vi "Rotate Two Files.vi"() -> ()   [LabVIEW 2021]
uses:
  6c21c491-3613-49b9-8739-58848ace7e6b.vi
  9d677228-37d7-4fae-91d8-cc659d765936.vi
  6babdee7-8c0c-47d0-81fc-a19b133f3013.vi
  911cfe7f-2ed1-4032-abb0-88a2fbac1f55.vi
panel:
  in  "Reverse File 2":bool
  in  "Averaging":dbl(slide) scale=1.0..1000.0
  in  "number of header lines":i32
  in  "Numeric":dbl step=5e-06 format="%.2e"
  out "X & Y 3":dbl[](graph)
  out "Array":sgl[](array[numeric]) format="%.2f"
  in  "Save":bool
  out "X & Y 2":dbl[][](graph)
  in  "CH2 File 1":sgl(slide) step=0.5 scale=-180.0..180.0
  in  "CH1 File 2":sgl(slide) step=0.1 scale=-180.0..180.0
  in  "CH2 File 2":sgl(slide) step=0.5 scale=-180.0..180.0
  in  "Channel 1 Y":i32=3
  in  "Channel 2 Y":i32=5
  in  "Channel 2 X":i32=4
  in  "Channel 1  X":i32=2
  out "X & Y":dbl[][](graph)
  in  "Phase OK":bool
  in  "CH1 File 1":sgl(slide) step=0.1 scale=-180.0..180.0
  in  "Input file 2":path
  in  "Data Source":T1(ring)
  in  "Input file 1":path
  # "ADD"
  # "ADD"
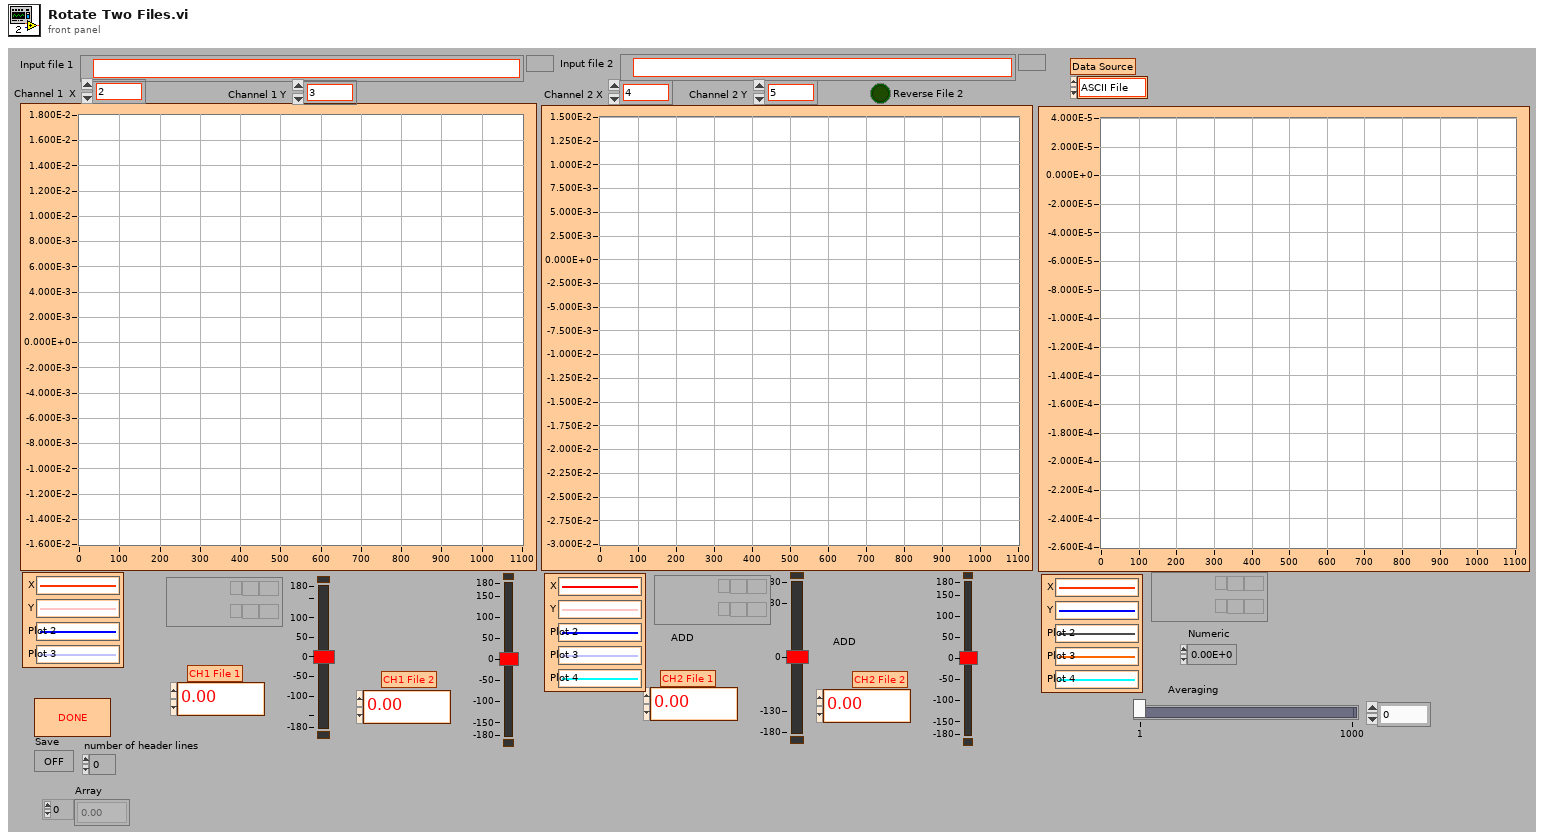
[diagram p1: front panel]
types:
  T1 = enum16{"ASCII File", "BinH File", "BinW File", "BINARY File"}
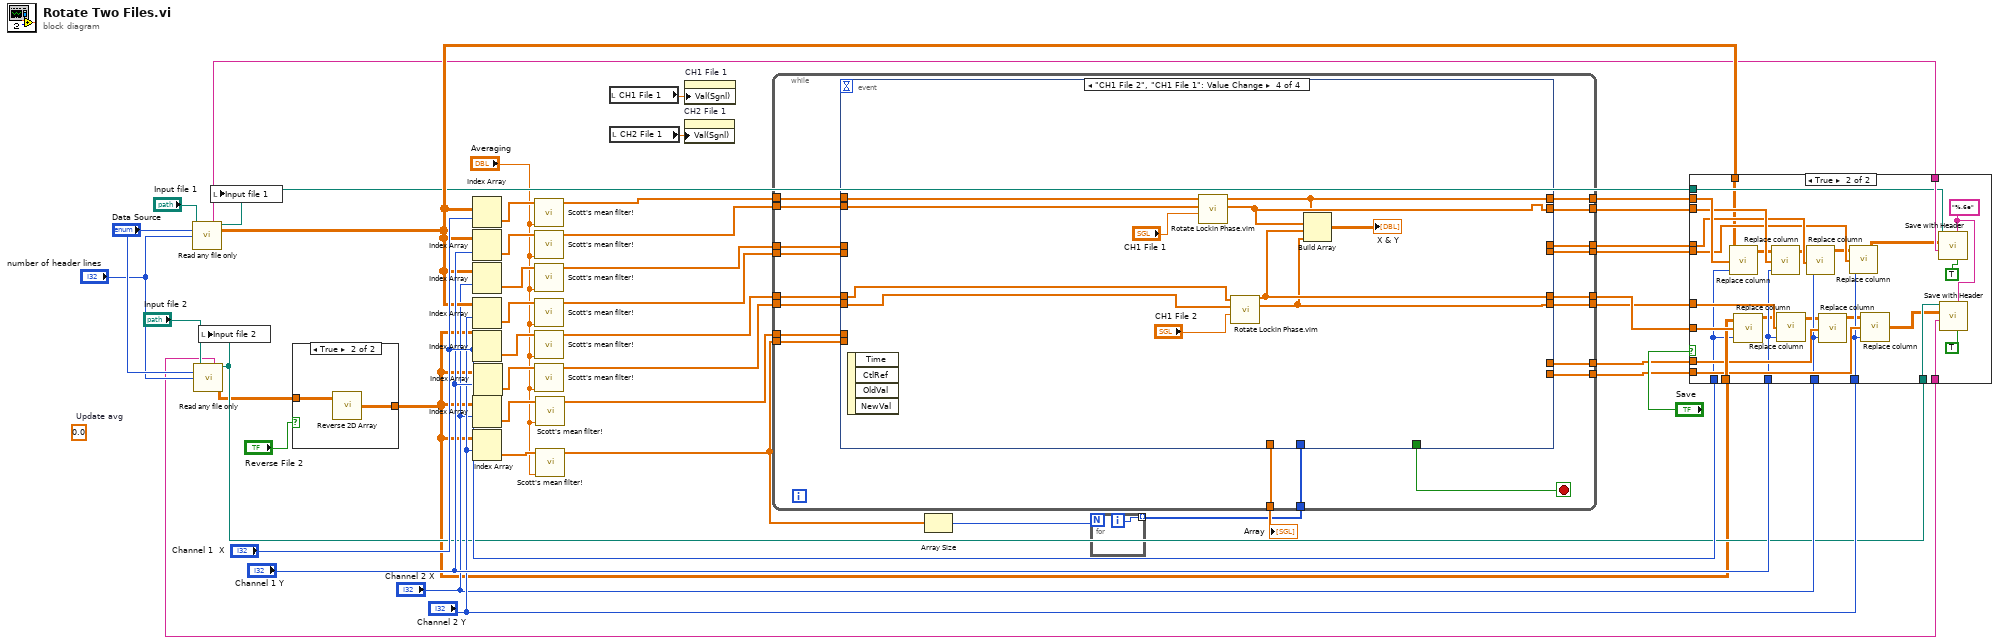
[diagram p0: block diagram]
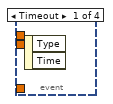
[diagram p3: hidden frame]
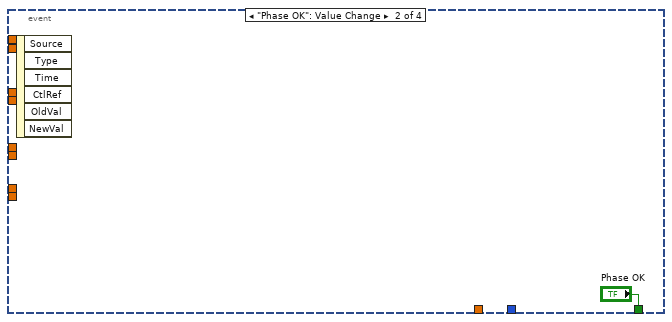
[diagram p4: hidden frame]
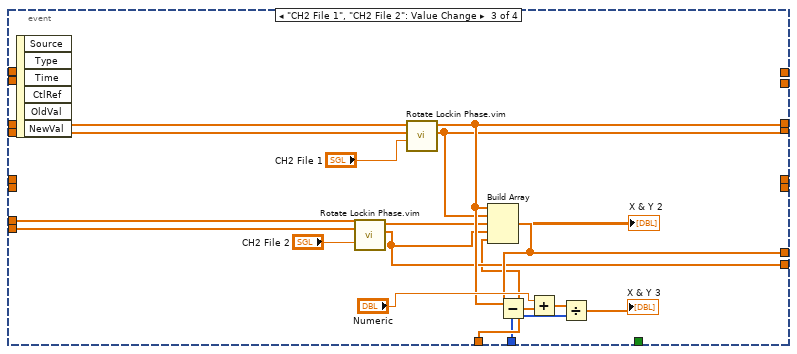
[diagram p5: hidden frame]
diagram:
  (unwired) 0.0  # Update avg
  n1 = call "Read any file only.vi"("Input file path"="Input file 1", "Data File Type"="Data Source", "number of header lines"="number of header lines") -> ("Header"=w26:string, "Actual input file path"=w24:path, "all rows"=w38:sgl[][])  [unwired: 6 in, 4 out]
  n2 = call "Read any file only.vi"("Input file path"="Input file 2", "Data File Type"="Data Source", "number of header lines"="number of header lines") -> ("Header"=w25:string, "Actual input file path"=w22:path, "all rows"=w2:sgl[][])  [unwired: 6 in, 4 out]
  n3 = local write "Input file 2"(w22) -> ()
  n4 = local write "Input file 1"(w24) -> ()
  n5 = case shown="True" "Reverse File 2" {
    tunnel: w2 -> [w48 w50]
    tunnel: [w48 w49] -> w1
    frame False {
    }
    frame True {
      n6 = call "Reverse 2D Array.vi"("Input array"=w50) -> ("Output Array"=w49:dbl[][])  [unwired: 1 in]
    }
  }
  n7 = Index Array(array=w38, index (row)="Channel 1  X") -> (element=w44:sgl[])  [unwired: 1 in]
  n8 = Index Array(array=w38, index (row)="Channel 1 Y") -> (element=w20:sgl[])  [unwired: 1 in]
  n9 = Index Array(array=w38, index (row)="Channel 2 X") -> (element=w18:sgl[])  [unwired: 1 in]
  n10 = Index Array(array=w38, index (row)="Channel 2 Y") -> (element=w16:sgl[])  [unwired: 1 in]
  n11 = Index Array(array=w1, index (row)="Channel 1  X") -> (element=w14:dbl[])  [unwired: 1 in]
  n12 = Index Array(array=w1, index (row)="Channel 2 X") -> (element=w10:dbl[])  [unwired: 1 in]
  n13 = Index Array(array=w1, index (row)="Channel 2 Y") -> (element=w8:dbl[])  [unwired: 1 in]
  n14 = Index Array(array=w1, index (row)="Channel 1 Y") -> (element=w12:dbl[])  [unwired: 1 in]
  n15 = call "Scott's mean filter!.vi"("window size"="Averaging", "input"=w44) -> ("output"=w21:dbl[])  [unwired: 9 out]
  n16 = call "Scott's mean filter!.vi"("window size"="Averaging", "input"=w20) -> ("output"=w19:dbl[])  [unwired: 9 out]
  n17 = call "Scott's mean filter!.vi"("window size"="Averaging", "input"=w18) -> ("output"=w17:dbl[])  [unwired: 9 out]
  n18 = call "Scott's mean filter!.vi"("window size"="Averaging", "input"=w16) -> ("output"=w15:dbl[])  [unwired: 9 out]
  n19 = call "Scott's mean filter!.vi"("window size"="Averaging", "input"=w14) -> ("output"=w13:dbl[])  [unwired: 9 out]
  n20 = call "Scott's mean filter!.vi"("window size"="Averaging", "input"=w12) -> ("output"=w11:dbl[])  [unwired: 9 out]
  n21 = call "Scott's mean filter!.vi"("window size"="Averaging", "input"=w10) -> ("output"=w9:dbl[])  [unwired: 9 out]
  n22 = call "Scott's mean filter!.vi"("window size"="Averaging", "input"=w8) -> ("output"=w7:dbl[])  [unwired: 9 out]
  n23 = local read "CH1 File 1"() -> (w4:sgl)
  n24 = local read "CH2 File 1"() -> (w5:sgl)
  n25 = property on="CH2 File 1" class="Slide (strict)"("Val(Sgnl)"=w5) -> ()  [unwired: 2 in, 2 out]
  n26 = property on="CH1 File 1" class="Slide (strict)"("Val(Sgnl)"=w4) -> ()  [unwired: 2 in, 2 out]
  n27 = Array Size(array=w7) -> (size(s)=w29:i32)
  n28 = for {
    N: w29 -> [_]
    tunnel: [w51] -> w28 mode=indexing
    i -> [w51]
  }
  n29 = while {
    tunnel: w28 -> [w55]
    tunnel: [w54] -> w30
    tunnel: [w57] -> w32
    tunnel: [w53] -> w33
    tunnel: [w58] -> w34
    tunnel: [w59] -> w35
    tunnel: [w60] -> w36
    tunnel: [w56] -> w37
    tunnel: [w61] -> w39
    tunnel: [w62] -> w40
    tunnel: w7 -> [w63]
    tunnel: w9 -> [w64]
    tunnel: w11 -> [w65]
    tunnel: w13 -> [w66]
    tunnel: w15 -> [w67]
    tunnel: w17 -> [w68]
    tunnel: w19 -> [w69]
    tunnel: w21 -> [w70]
    stop <- w52 stop-if-true
    n30 = event shown="[3] \"CH1 File 2\", \"CH1 File 1\": Value Change" {
      selector: _ -> [_ _ _ _]
      dyn-events: _ -> [_ _ _ _]
      timeout: _ -> [_ _ _ _]
      tunnel: w70 -> [_ _ _ w91]
      tunnel: w69 -> [_ _ _ w90]
      tunnel: w68 -> [_ _ w76 _]
      tunnel: w67 -> [_ _ w75 _]
      tunnel: w66 -> [_ _ _ w89]
      tunnel: w65 -> [_ _ _ w88]
      tunnel: w64 -> [_ _ w74 _]
      tunnel: w63 -> [_ _ w73 _]
      tunnel: [_ _ _ w95] -> w62
      tunnel: [_ _ _ w96] -> w61
      tunnel: [_ _ w81 _] -> w60
      tunnel: [_ _ _ w93] -> w59
      tunnel: [_ _ _ w92] -> w58
      tunnel: [_ _ w79 _] -> w57
      tunnel: [_ _ w82 _] -> w56
      tunnel: w55 -> [_ _ w77 _]
      tunnel: [_ _ w78 _] -> w54
      tunnel: [_ _ w80 _] -> w53
      tunnel: [_ "Phase OK" _ _] -> w52
      event Timeout {
        n31 = event-data() -> ()  [unwired: 3 out]
      }
      event "Phase OK": Value Change {
        n32 = event-data() -> ()  [unwired: 7 out]
      }
      event "CH2 File 1", "CH2 File 2": Value Change {
        n33 = event-data() -> ()  [unwired: 7 out]
        n34 = call "Rotate Lockin Phase.vim"("Phase"="CH2 File 2", "Array Y in"=w73, "Array X in"=w74) -> ("Array Y out"=w79:dbl[], "Array X out"=w80:dbl[])  [unwired: 7 in]
        n35 = call "Rotate Lockin Phase.vim"("Phase"="CH2 File 1", "Array Y in"=w75, "Array X in"=w76) -> ("Array Y out"=w81:dbl[], "Array X out"=w82:dbl[])  [unwired: 7 in]
        n36 = Subtract(x=w82, y=w80) -> (x-y=w78:dbl[])
        n37 = Build Array(w82, w81, w80, w79, w78) -> (→"X & Y 2":dbl[][])
        n38 = Add(x="Numeric", y=w78) -> (x+y=w84:dbl[])
        n39 = Divide(x=w84, y=w77) -> (x/y=→"X & Y 3":dbl[])
      }
      event "CH1 File 2", "CH1 File 1": Value Change {
        n40 = event-data() -> ()  [unwired: 5 out]
        n41 = call "Rotate Lockin Phase.vim"("Phase"="CH1 File 1", "Array Y in"=w90, "Array X in"=w91) -> ("Array Y out"=w96:dbl[], "Array X out"=w95:dbl[])  [unwired: 7 in]
        n42 = call "Rotate Lockin Phase.vim"("Phase"="CH1 File 2", "Array Y in"=w88, "Array X in"=w89) -> ("Array Y out"=w92:dbl[], "Array X out"=w93:dbl[])  [unwired: 7 in]
        n43 = Build Array(w95, w96, w93, w92) -> (→"X & Y":dbl[][])
      }
    }
  }
  "Array" <- w30
  n44 = case shown="True" "Save" {
    tunnel: "Channel 1  X" -> [_ w118]
    tunnel: "Channel 1 Y" -> [_ w117]
    tunnel: w40 -> [_ w127]
    tunnel: w39 -> [_ w126]
    tunnel: w38 -> [_ w102]
    tunnel: w37 -> [_ w125]
    tunnel: w36 -> [_ w124]
    tunnel: w1 -> [_ w122]
    tunnel: w35 -> [_ w123]
    tunnel: w34 -> [_ w121]
    tunnel: w33 -> [_ w120]
    tunnel: w32 -> [_ w119]
    tunnel: "Channel 2 X" -> [_ w115]
    tunnel: "Channel 2 Y" -> [_ w116]
    tunnel: w26 -> [_ w114]
    tunnel: w25 -> [_ w113]
    tunnel: w24 -> [_ w111]
    tunnel: w22 -> [_ w110]
    frame False {
    }
    frame True {
      w112 = "%.6e" ("format (%.3f)")
      n45 = call "Replace column.vi"("Column index"=w118, "Column"=w127, "Input array"=w102) -> ("Output array"=w101:sgl[][])
      n46 = call "Replace column.vi"("Column index"=w118, "Column"=w123, "Input array"=w122) -> ("Output array"=w105:sgl[][])
      n47 = call "Replace column.vi"("Column index"=w117, "Column"=w126, "Input array"=w101) -> ("Output array"=w100:sgl[][])
      n48 = call "Replace column.vi"("Column index"=w117, "Column"=w121, "Input array"=w105) -> ("Output array"=w104:sgl[][])
      n49 = call "Replace column.vi"("Column index"=w115, "Column"=w125, "Input array"=w100) -> ("Output array"=w99:sgl[][])
      n50 = call "Replace column.vi"("Column index"=w115, "Column"=w120, "Input array"=w104) -> ("Output array"=w103:sgl[][])
      n51 = call "Replace column.vi"("Column index"=w116, "Column"=w124, "Input array"=w99) -> ("Output array"=w108:sgl[][])
      n52 = call "Replace column.vi"("Column index"=w116, "Column"=w119, "Input array"=w103) -> ("Output array"=w109:sgl[][])
      n53 = call "Save with Header.vi"("transpose? (no:F)"=TRUE, "format (%.3f)"=w112, "Header"=w114, "2D data"=w108, "file path (dialog if empty)"=w111) -> ()  [unwired: 7 out]
      n54 = call "Save with Header.vi"("transpose? (no:F)"=TRUE, "format (%.3f)"=w112, "Header"=w113, "2D data"=w109, "file path (dialog if empty)"=w110) -> ()  [unwired: 7 out]
    }
  }
